vi "two action by one queue.vi"() -> ()   [LabVIEW 2017]
uses:
  tools/queue/subvi/initSingle.vi
  tools/queue/subvi/readSingle.vi
  tools/queue/subvi/dataUnpackBool.vi
  tools/queue/subvi/sendSingle.vi
panel:
  in  "停止":bool
  in  "B":bool
  in  "A":bool
  out "B_action":bool=TRUE
  out "B_action":string
  out "A_action":bool=TRUE
  out "A_action":string
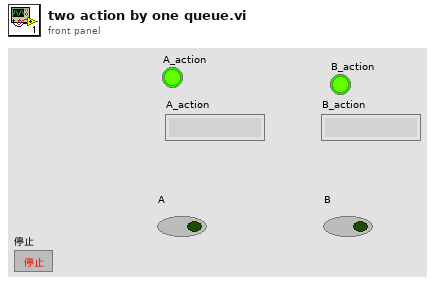
[diagram p1: front panel]
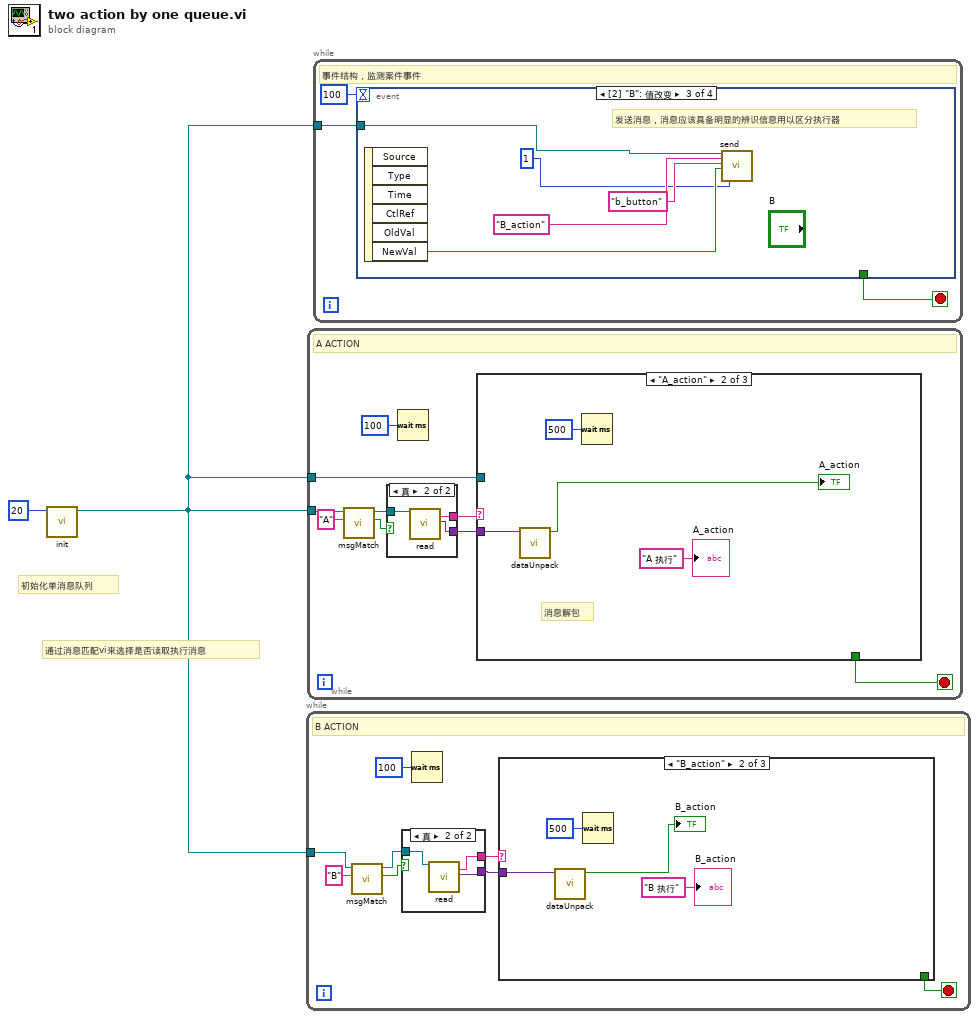
[diagram p0: block diagram]
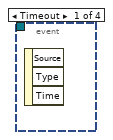
[diagram p2: hidden frame]
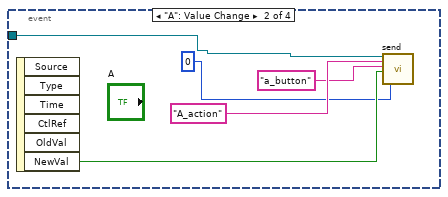
[diagram p3: hidden frame]
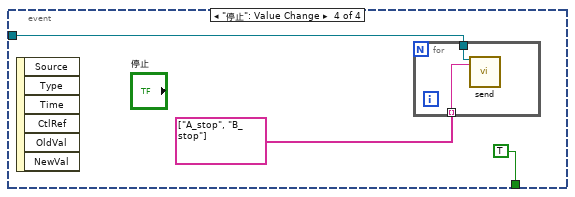
[diagram p4: hidden frame]
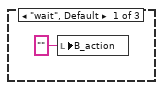
[diagram p6: hidden frame]
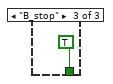
[diagram p7: hidden frame]
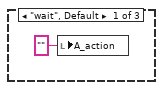
[diagram p9: hidden frame]
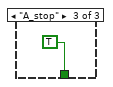
[diagram p10: hidden frame]
diagram:
  # "通过消息匹配vi来选择是否读取执行消息"
  # "初始化单消息队列"
  n1 = call-poly "init.vi"("size(-1)"=20) -> ("refer"=w1:refnum<queue>)  [unwired: 9 in, 1 out]
  n2 = while {
    tunnel: w1 -> [w6]
    stop <- w8 stop-if-true
    # "B ACTION"
    n3 = call "msgMatch.vi"("msgMatcher"="B", "refer"=w6) -> ("match"=w3:bool, "refer"=w4:refnum<queue>)  [unwired: 7 in, 1 out]
    n4 = case shown="真" w3 {
      tunnel: [_ w11] -> w9
      tunnel: [_ w12] -> w7
      tunnel: w4 -> [_ w13]
      frame False {
      }
      frame True {
        n5 = call-poly "read.vi"("refer"=w13) -> ("to"=w11:string, "data"=w12:variant)  [unwired: 11 in, 6 out]
      }
    }
    n6 = Wait (ms)(milliseconds to wait=u32 100 ("等待时间（毫秒）")) -> ()  [unwired: 1 out]
    n7 = case shown="\"B_action\"" w9 {
      tunnel: [_ _ TRUE] -> w8
      tunnel: w7 -> [_ w16 _]
      frame "wait", Default {
        n8 = local write "B_action"("" ("B_action")) -> ()
      }
      frame "B_action" {
        n9 = call-poly "dataUnpack.vi"("data"=w16) -> ("bool"=→"B_action":bool)  [unwired: 9 in, 1 out]
        n10 = Wait (ms)(milliseconds to wait=u32 500 ("等待时间（毫秒）")) -> ()  [unwired: 1 out]
        "B_action" <- "B 执行" ("B_action")
      }
      frame "B_stop" {
      }
    }
  }
  n11 = while {
    tunnel: w1 -> [w25]
    tunnel: w1 -> [w20]
    stop <- w27 stop-if-true
    # "A ACTION"
    n12 = call "msgMatch.vi"("msgMatcher"="A", "refer"=w25) -> ("match"=w22:bool, "refer"=w23:refnum<queue>)  [unwired: 7 in, 1 out]
    n13 = case shown="真" w22 {
      tunnel: [_ w30] -> w26
      tunnel: w23 -> [_ w31]
      tunnel: [_ w29] -> w21
      frame False {
      }
      frame True {
        n14 = call-poly "read.vi"("refer"=w31) -> ("to"=w29:string, "data"=w30:variant)  [unwired: 11 in, 6 out]
      }
    }
    n15 = Wait (ms)(milliseconds to wait=u32 100 ("等待时间（毫秒）")) -> ()  [unwired: 1 out]
    n16 = case shown="\"A_action\"" w21 {
      tunnel: [_ _ TRUE] -> w27
      tunnel: w26 -> [_ w34 _]
      tunnel: w20 -> [_ _ _]
      frame "wait", Default {
        n17 = local write "A_action"("" ("A_action")) -> ()
      }
      frame "A_action" {
        # "消息解包"
        n18 = call-poly "dataUnpack.vi"("data"=w34) -> ("bool"=→"A_action":bool)  [unwired: 9 in, 1 out]
        n19 = Wait (ms)(milliseconds to wait=u32 500 ("等待时间（毫秒）")) -> ()  [unwired: 1 out]
        "A_action" <- "A 执行" ("A_action")
      }
      frame "A_stop" {
      }
    }
  }
  n20 = while {
    tunnel: w1 -> [w39]
    stop <- w38 stop-if-true
    # "事件结构，监测案件事件"
    n21 = event shown="[2] \"B\": 值改变" {
      selector: _ -> [_ _ _ _]
      dyn-events: _ -> [_ _ _ _]
      timeout: 100 -> [_ _ _ _]
      tunnel: w39 -> [_ w42 w47 w51]
      tunnel: [_ _ _ TRUE] -> w38
      event Timeout {
        n22 = event-data() -> ()  [unwired: 1 in, 3 out]
      }
      event "A": Value Change {
        n23 = event-data() -> ("NewVal"=w43:bool)  [unwired: 1 in, 5 out]
        n24 = call-poly "send.vi"("refer"=w42, "to"="A_action", "from"="a_button", "data"=w43, "index"=0 ("Index")) -> ()  [unwired: 13 in, 2 out]
      }
      event "B": Value Change {
        # "发送消息，消息应该具备明显的辨识信息用以区分执行器"
        n25 = event-data() -> ("NewVal"=w48:bool)  [unwired: 1 in, 5 out]
        n26 = call-poly "send.vi"("refer"=w47, "to"="B_action" ("to 2"), "from"="b_button", "data"=w48, "index"=1 ("Index")) -> ()  [unwired: 13 in, 2 out]
      }
      event "停止": Value Change {
        n27 = event-data() -> ()  [unwired: 1 in, 6 out]
        n28 = for {
          tunnel: string[] ["A_stop", "B_stop"] ("to 2") -> [w55] mode=indexing
          tunnel: w51 -> [w54]
          n29 = call-poly "send.vi"("refer"=w54, "to"=w55) -> ()  [unwired: 16 in, 2 out]
        }
      }
    }
  }
